vi "IMIC_GetXSpeedProp.vi"(3 "Enum":T1(ring)=enum."max", 5 "handle":u64) -> (0 "Property":dbl, 1 "handle out":u64, 2 "output param":T2(ring))   [LabVIEW 2011]
uses:
  tillimic64.dll
panel:
  # "never used"
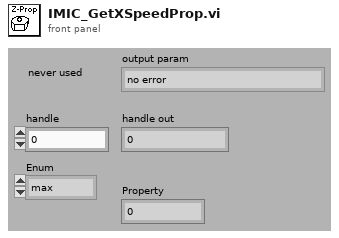
[diagram p1: front panel]
types:
  T1 = enum32{"min", "resolution", "max", "no property"}
  T2 = enum16{"no error", "missing axis", "missing Z axis", "missing Filter", "iMic not initialized", "no property", "wrong handle", "protocol not finished", "user parameter to long (>32 bits)", "no user parameter handle", "failed to open comport", "failed to initialize"}
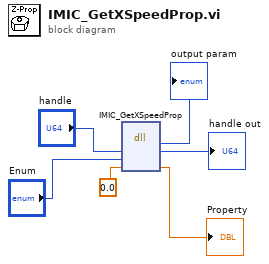
[diagram p0: block diagram]
diagram:
  n1 = dll-call lib="C:/Program Files/colibri/Drivers/TILLPhotonics/tillimic*.*" fn="IMIC_GetXSpeedProp"("handle"="handle", "propindex"="Enum", "propValue"=0.0) -> ("return type"=→"output param":i32, "handle"=→"handle out":u64, "propValue"=→"Property":dbl)  [unwired: 4 in, 2 out]
